vi "Write Filter Error Limits.vi"(8 "error in (no error)":errorcluster, 10 "Filter Error Limits (+/- V)":dbl=0.06, 11 "Frequency Measurement in":refnum<class "Frequency Measurement.lvclass">) -> (0 "error out":errorcluster, 3 "Frequency Measurement out":refnum<class "Frequency Measurement.lvclass">)   [LabVIEW 2013, in "Frequency Measurement.lvlib" / "Frequency Measurement.lvclass"]
uses:
  Frequency Measurement.lvclass
  Frequency Measurement.lvclass/Frequency Measurement.ctl
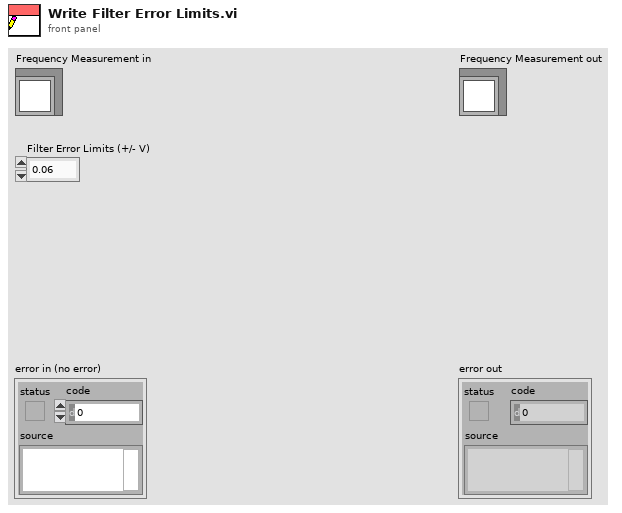
[diagram p1: front panel]
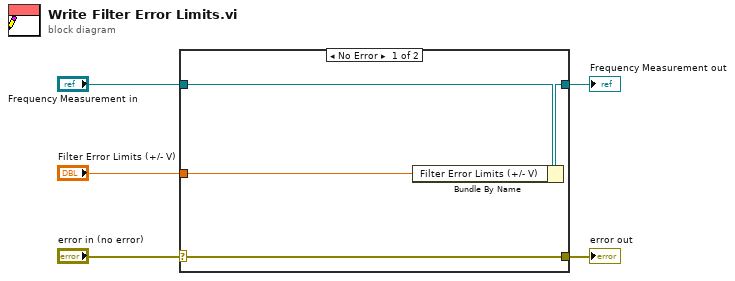
[diagram p0: block diagram]
diagram:
  n1 = case shown="No Error" "error in (no error)" {
    selector: "error in (no error)" -> [w9 w10]
    tunnel: [w9 w10] -> w4
    tunnel: [w7 w11] -> w2
    tunnel: "Frequency Measurement in" -> [w8 w11]
    tunnel: "Filter Error Limits (+/- V)" -> [w6 _]
    frame No Error {
      n2 = Bundle By Name(cluster=w8, "Filter Error Limits (+/- V)"=w6) -> (w7:refnum<class "Frequency Measurement.lvclass">)
    }
    frame Error {
    }
  }
  "error out" <- w4
  "Frequency Measurement out" <- w2
